vi "Handle Local Error.vi"(8 "Error In":errorcluster) -> (0 "Error Out":errorcluster)   [LabVIEW 2023, in "Error Manager.lvlib" / "New Error Dialogue GUI.lvlib"]
doc: "If the \"Error In\" input contains \"No Error\" this VI does nothing.\nIf the \"Error In\" input contains an error this VI:\n1. Enqueues the \"Local Error Handler\" command, with the \"Error In\" error as the message data\n2. Clears the error. This guarantees that the \"Error Out\" output of this VI always contains \"No Error\"."
uses:
  New Error Dialogue GUI.lvlib
  MHL Queue/Command (enum).ctl
  MHL Queue/MHL Queue.lvlib
panel:
  # "Development\ncontrols/indicators useful for development and testing, but which are not outputs of the VI"
  # "Input\nInputs to the VI"
  # "Output\nOutputs of the VI"
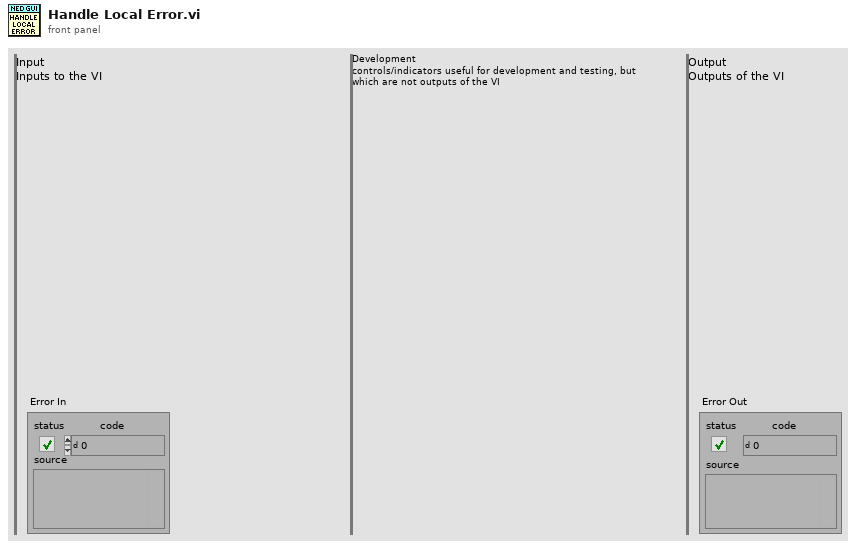
[diagram p1: front panel]
types:
  T1 = typedef "Error Manager.lvlib/New Error Dialogue GUI.lvlib/MHL Queue.lvlib/Command (enum).ctl" = enum16{"Init Module", "Close Module", "Handle Local Error", "OK Button Pressed"}
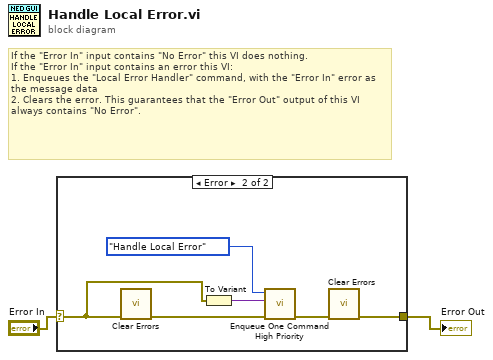
[diagram p0: block diagram]
diagram:
  # "If the \"Error In\" input contains \"No Error\" this VI does nothing.\nIf the \"Error In\" input contains an error this VI:\n1. Enqueues the \"Local Error Handler\" command, with the \"Error In\" error as the message data\n2. Clears the error. This guarantees that the \"Error Out\" output of this VI always contains \"No Error\"."
  n1 = case shown="Error" "Error In" {
    selector: "Error In" -> [w3 w8]
    tunnel: [w3 w5] -> w1
    frame No Error {
      # "Do nothing if there is \"No Error\" at input."
    }
    frame Error {
      n2 = call <vilib>:"Clear Errors.vi"("error in (no error)"=w8) -> ("error out"=w7:errorcluster)  [unwired: 5 in, 1 out]
      n3 = To Variant(anything=w8) -> (Variant=w9:variant)
      n4 = call "Enqueue One Command High Priority.vi"("error in (no error)"=w7, "Data"=w9, "Command"=Command_(enum)."Handle Local Error") -> ("error out"=w6:errorcluster)  [unwired: 8 in]
      n5 = call <vilib>:"Clear Errors.vi"("error in (no error)"=w6) -> ("error out"=w5:errorcluster)  [unwired: 5 in, 1 out]
    }
  }
  "Error Out" <- w1
